vi "AB_RW_Project_Source_RESTfulVI.vi"(7 "action":T7, 8 "error in (no error)":errorcluster, 9 "index in":i32, 10 "dataSource in":T1={"RESTful VI configuration"={"Service VI Type"=enum."Web Method", "Load VI at statup"=TRUE, "Keep VI in memory"=TRUE, "Output type"=enum."Terminal", "Output format"=enum."XML", "Use headers"=TRUE, "Buffered"=TRUE, "eng_Load VI by name"=FALSE}}, 11 "buildObject":T6) -> (0 "error out":errorcluster, 1 "index out":i32, 2 "dataSource out":T1={"RESTful VI configuration"={"Service VI Type"=enum."Web Method", "Load VI at statup"=TRUE, "Keep VI in memory"=TRUE, "Output type"=enum."Terminal", "Output format"=enum."XML", "Use headers"=TRUE, "Buffered"=TRUE, "eng_Load VI by name"=FALSE}}, 3 "buildObject out":T6)   [LabVIEW 2020]
doc: "Reads and writes the data to the object property bag."
uses:
  <resource>/Framework/Providers/API/ItemRef.ctl
  <vilib>/AppBuilder/RW_Project/AB_RW_Project_PropBag_Action.ctl
  <vilib>/AppBuilder/RW_Project/AB_RW_Project_Source_RESTfulVI_Data.ctl
  <vilib>/AppBuilder/AB_Classes/Source/RESTfulVI/Configure_RESTfulVI/AB_RESTful_Configuration.ctl
  <vilib>/AppBuilder/AB_Classes/Source/RESTfulVI/Configure_RESTfulVI/AB_RESTful_VIType.ctl
  <vilib>/AppBuilder/AB_Classes/Source/RESTfulVI/Configure_RESTfulVI/AB_RESTful_OutputType.ctl
  <vilib>/AppBuilder/AB_Classes/Source/RESTfulVI/Configure_RESTfulVI/AB_RESTful_OutputFormat.ctl
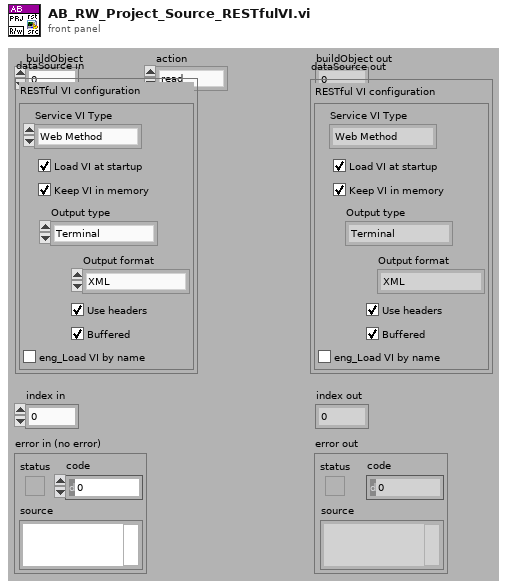
[diagram p1: front panel]
types:
  T1 = typedef "AB_RW_Project_Source_RESTfulVI_Data.ctl" = cluster{"RESTful VI configuration":T2}
  T2 = typedef "AB_RESTful_Configuration.ctl" = cluster{"Service VI Type":T3, "Load VI at statup":bool, "Keep VI in memory":bool, "Output type":T4, "Output format":T5, "Use headers":bool, "Buffered":bool, "eng_Load VI by name":bool}
  T3 = typedef "AB_RESTful_VIType.ctl" = enum32{"Web Method", "Auxiliary", "eng_Internal", "eng_Content"}
  T4 = typedef "AB_RESTful_OutputType.ctl" = enum32{"Terminal", "Stream"}
  T5 = typedef "AB_RESTful_OutputFormat.ctl" = enum32{"XML", "Text", "HTML", "JSON"}
  T6 = typedef "ItemRef.ctl" = u64
  T7 = typedef "AB_RW_Project_PropBag_Action.ctl" = enum16{"read", "write", "clear", "readPrevious", "writePrevious", "clearPrevious"}
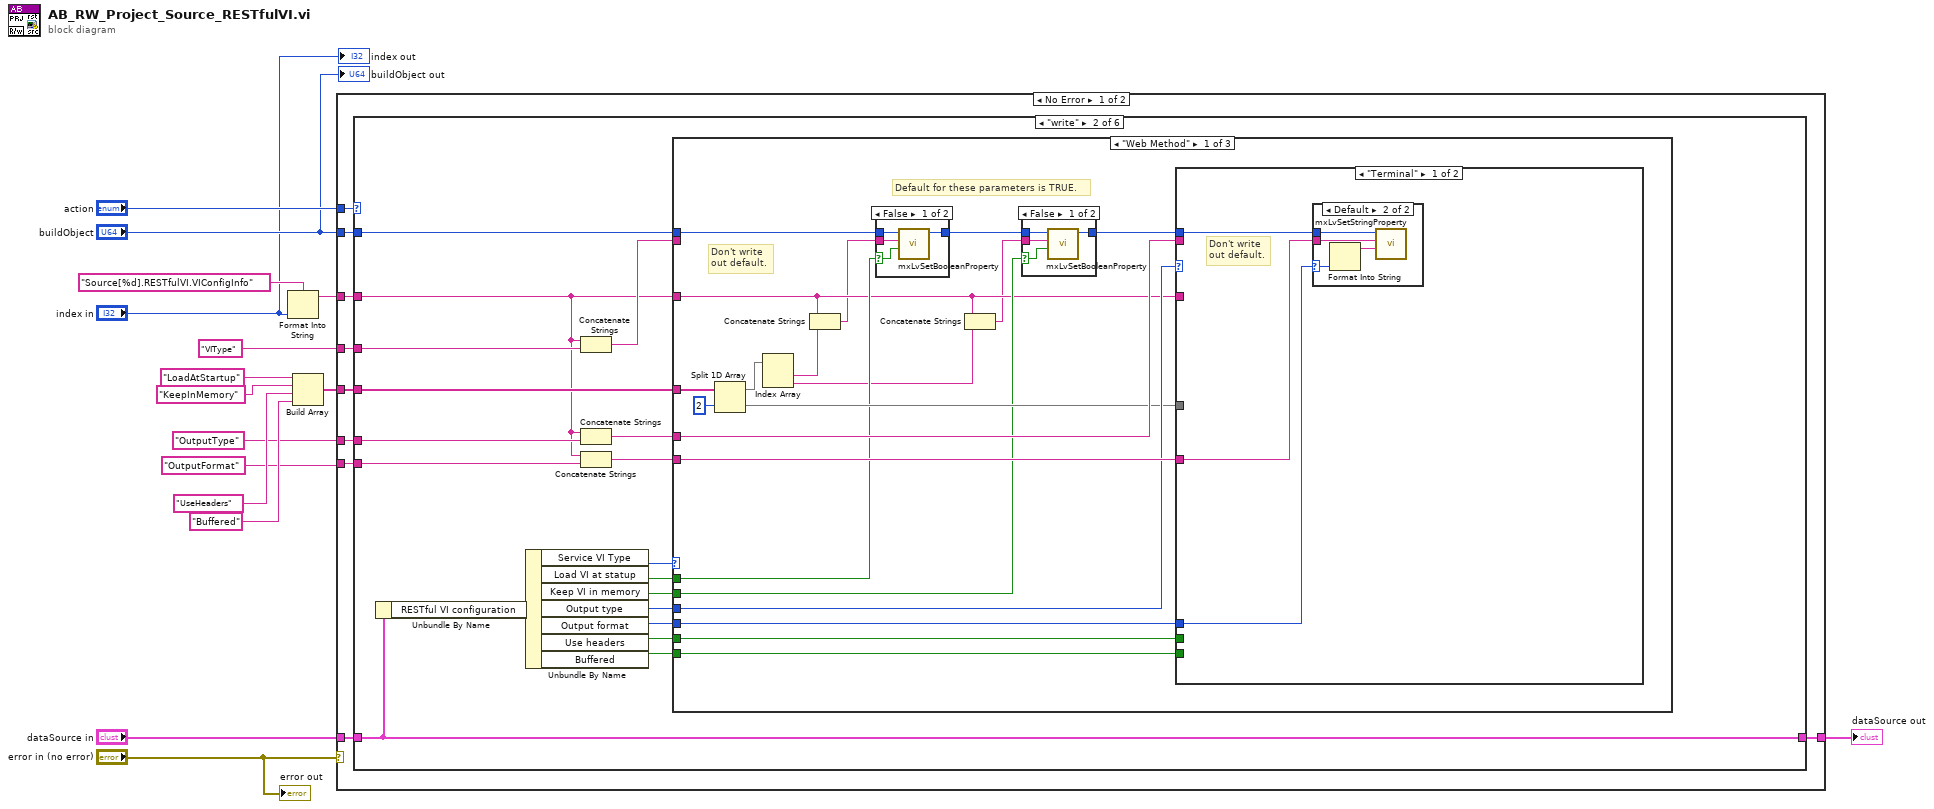
[diagram p0: block diagram]
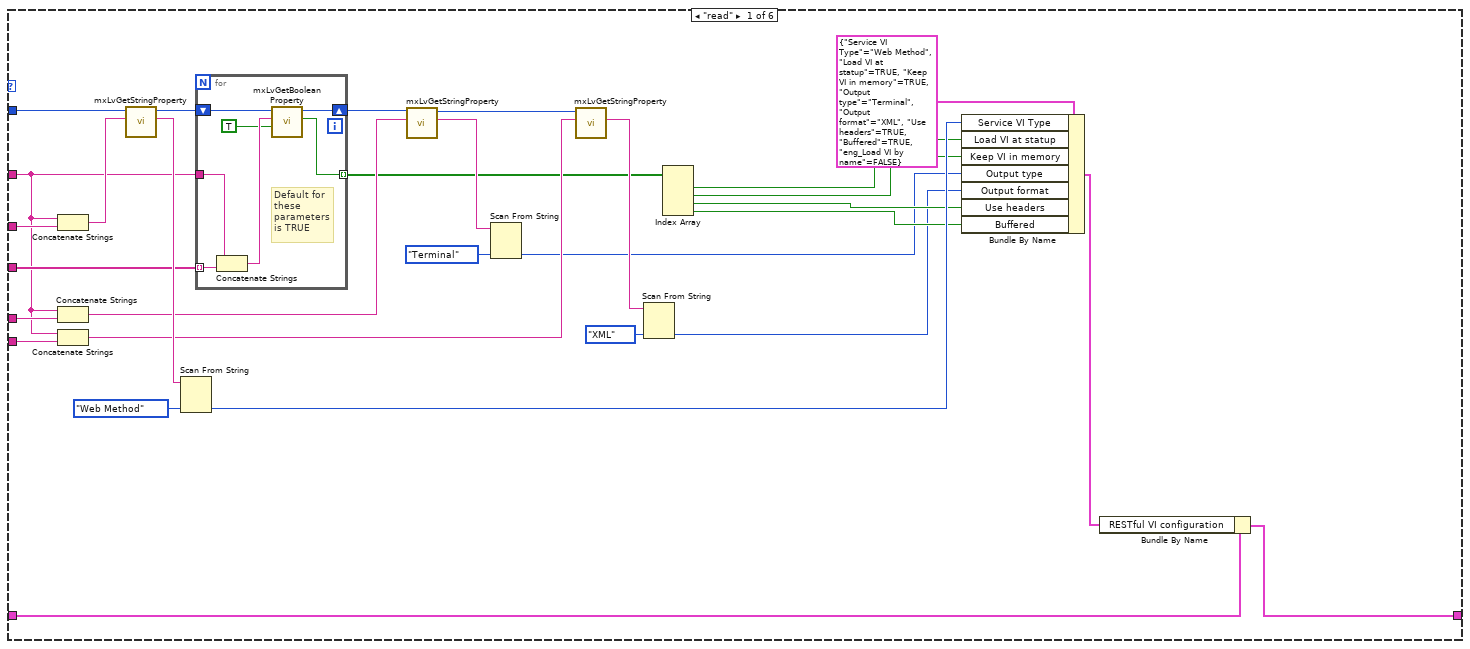
[diagram p2: hidden frame]
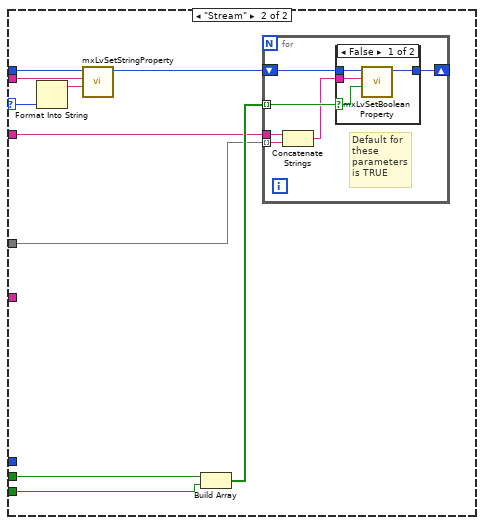
[diagram p6: hidden frame]
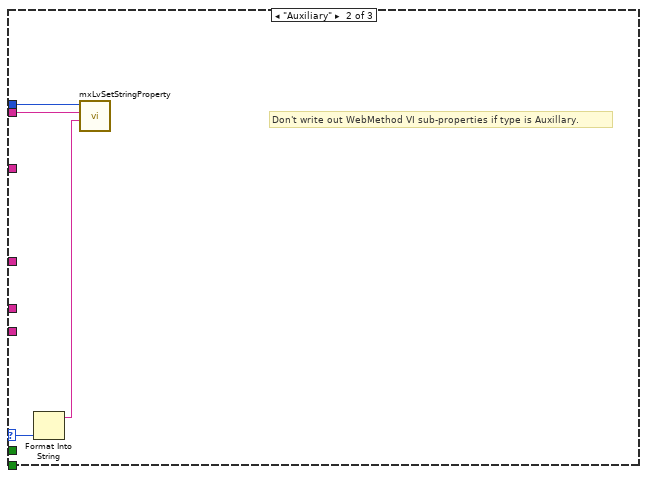
[diagram p8: hidden frame]
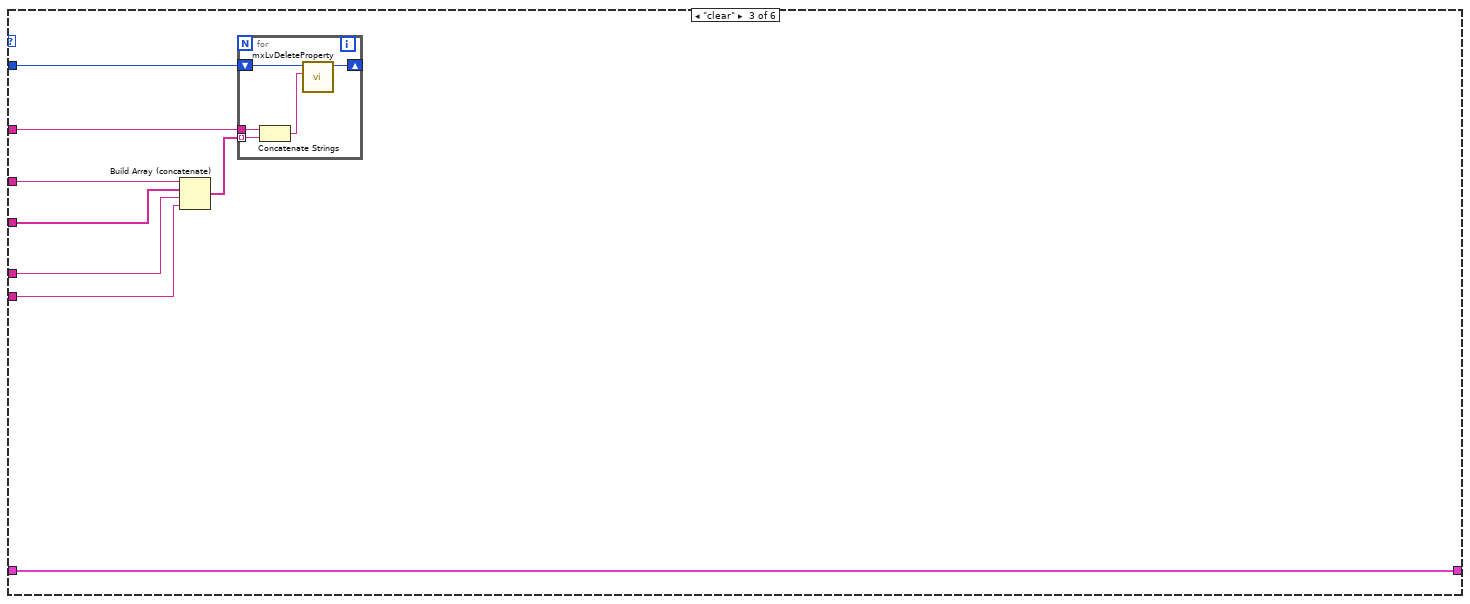
[diagram p10: hidden frame]
diagram:
  n1 = Format Into String(format string="Source[%d].RESTfulVI.VIConfigInfo", "index in") -> (resulting string=w14:string)  [unwired: 2 in, 1 out]
  n2 = Build Array("LoadAtStartup", "KeepInMemory", "UseHeaders", "Buffered") -> (w2:string[])
  n3 = case shown="No Error" "error in (no error)" {
    tunnel: "action" -> [w25 _]
    tunnel: "dataSource in" -> [w24 w159]
    tunnel: w14 -> [w23 _]
    tunnel: "buildObject" -> [w22 _]
    tunnel: [w21 w159] -> w9
    tunnel: "VIType" -> [w20 _]
    tunnel: "OutputType" -> [w19 _]
    tunnel: "OutputFormat" -> [w18 _]
    tunnel: w2 -> [w17 _]
    frame No Error {
      n4 = case shown="\"write\"" w25 {
        tunnel: w22 -> [w50 w78 w149 _ _ _]
        tunnel: w24 -> [w55 w80 w150 w156 w157 w158]
        tunnel: w23 -> [w42 w64 w144 _ _ _]
        tunnel: [w54 w80 w150 w156 w157 w158] -> w21
        tunnel: w20 -> [w51 w77 w147 _ _ _]
        tunnel: w19 -> [w43 w70 w146 _ _ _]
        tunnel: w18 -> [w41 w69 w145 _ _ _]
        tunnel: w17 -> [w45 w71 w148 _ _ _]
        frame "read" {
          n5 = Concatenate Strings(w42, w51) -> (w49:string)
          n6 = Concatenate Strings(w42, w43) -> (w39:string)
          n7 = Concatenate Strings(w42, w41) -> (w37:string)
          n8 = call <resource>:"mxLvGetStringProperty.vi"("Tag"=w49, "Item"=w50) -> ("Value"=w48:string, "Item"=w44:T6)  [unwired: 1 in, 7 out]
          n9 = Scan From String(input string=w48, default 1=AB_RESTful_VIType."Web Method" ("Service VI Type")) -> (output 1=w46:T3)  [unwired: 3 in, 3 out]
          n10 = for {
            tunnel: w45 -> [w61] mode=indexing
            tunnel: w42 -> [w62]
            shift-right: [w59] -> w40
            shift-left: w44 -> [w60]
            tunnel: [w57] -> w32 mode=indexing
            # "Default for these parameters is TRUE"
            n11 = Concatenate Strings(w62, w61) -> (w58:string)
            n12 = call <resource>:"mxLvGetBooleanProperty.vi"("Default Value (F)"=TRUE, "Tag"=w58, "Item"=w60) -> ("Value"=w57:bool, "Item"=w59:T6)  [unwired: 1 in, 6 out]
          }
          n13 = call <resource>:"mxLvGetStringProperty.vi"("Tag"=w39, "Item"=w40) -> ("Value"=w36:string, "Item"=w38:T6)  [unwired: 1 in, 7 out]
          n14 = Scan From String(input string=w36, default 1=AB_RESTful_OutputType."Terminal" ("Output type")) -> (output 1=w26:T4)  [unwired: 3 in, 3 out]
          n15 = call <resource>:"mxLvGetStringProperty.vi"("Tag"=w37, "Item"=w38) -> ("Value"=w34:string)  [unwired: 1 in, 8 out]
          n16 = Scan From String(input string=w34, default 1=AB_RESTful_OutputFormat."XML" ("Output format")) -> (output 1=w27:T5)  [unwired: 3 in, 3 out]
          n17 = Index Array(array=w32) -> (element #1=w31:bool, element #2=w30:bool, element #3=w29:bool, element #4=w28:bool)  [unwired: 4 in]
          n18 = Bundle By Name(cluster=T2 {"Service VI Type"=enum."Web Method", "Load VI at statup"=TRUE, "Keep VI in memory"=TRUE, "Output type"=enum."Terminal", "Output format"=enum."XML", "Use headers"=TRUE, "Buffered"=TRUE, "eng_Load VI by name"=FALSE} ("RESTful VI configuration"), "Service VI Type"=w46, "Load VI at statup"=w31, "Keep VI in memory"=w30, "Output type"=w26, "Output format"=w27, "Use headers"=w29, "Buffered"=w28) -> (w53:T2)
          n19 = Bundle By Name(cluster=w55, "RESTful VI configuration"=w53) -> (w54:T1)
        }
        frame "write" {
          n20 = Unbundle By Name(w80) -> ("RESTful VI configuration"=w79:T2)
          n21 = Unbundle By Name(w79) -> ("Service VI Type"=w63:T3, "Load VI at statup"=w75:bool, "Keep VI in memory"=w74:bool, "Output type"=w66:T4, "Output format"=w65:T5, "Use headers"=w73:bool, "Buffered"=w72:bool)
          n22 = Concatenate Strings(w64, w77) -> (w76:string)
          n23 = Concatenate Strings(w64, w70) -> (w68:string)
          n24 = Concatenate Strings(w64, w69) -> (w67:string)
          n25 = case shown="\"Web Method\"" w63 {
            selector: w63 -> [_ w139 _]
            tunnel: w78 -> [w91 w141 _]
            tunnel: w76 -> [_ w140 _]
            tunnel: w75 -> [w88 _ _]
            tunnel: w74 -> [w87 _ _]
            tunnel: w73 -> [w100 _ _]
            tunnel: w72 -> [w99 _ _]
            tunnel: w71 -> [w93 _ _]
            tunnel: w68 -> [w98 _ _]
            tunnel: w67 -> [w97 _ _]
            tunnel: w66 -> [w95 _ _]
            tunnel: w65 -> [w96 _ _]
            tunnel: w64 -> [w85 _ _]
            frame "Web Method" {
              # "Default for these parameters is TRUE."
              # "Don't write out default."
              n26 = Split 1D Array(array=w93, index=2) -> (first subarray=w86:string[], second subarray=w92:string[])
              n27 = Index Array(array=w86) -> (element #1=w84:string, element #2=w82:string)  [unwired: 2 in]
              n28 = Concatenate Strings(w85, w84) -> (w83:string)
              n29 = case shown="False" w88 {
                selector: w88 -> [w107 _]
                tunnel: w91 -> [w109 w110]
                tunnel: [w108 w110] -> w90
                tunnel: w83 -> [w106 _]
                frame False {
                  n30 = call <resource>:"mxLvSetBooleanProperty.vi"("Value (F)"=w107, "Tag"=w106, "Item"=w109) -> ("Item"=w108:T6)  [unwired: 2 in, 6 out]
                }
                frame True {
                }
              }
              n31 = Concatenate Strings(w85, w82) -> (w81:string)
              n32 = case shown="False" w87 {
                selector: w87 -> [w102 _]
                tunnel: w90 -> [w104 w105]
                tunnel: [w103 w105] -> w89
                tunnel: w81 -> [w101 _]
                frame False {
                  n33 = call <resource>:"mxLvSetBooleanProperty.vi"("Value (F)"=w102, "Tag"=w101, "Item"=w104) -> ("Item"=w103:T6)  [unwired: 2 in, 6 out]
                }
                frame True {
                }
              }
              n34 = case shown="\"Terminal\"" w95 {
                selector: w95 -> [_ w118]
                tunnel: w100 -> [_ w127]
                tunnel: w99 -> [_ w126]
                tunnel: w92 -> [_ w124]
                tunnel: w98 -> [_ w122]
                tunnel: w97 -> [w113 _]
                tunnel: w96 -> [w112 _]
                tunnel: w85 -> [_ w121]
                tunnel: w89 -> [w111 w120]
                frame "Terminal" {
                  # "Don't write out default."
                  n35 = case shown="Default" w112 {
                    selector: w112 -> [_ w114]
                    tunnel: w111 -> [_ w117]
                    tunnel: w113 -> [_ w115]
                    frame "XML" {
                    }
                    frame Default {
                      n36 = Format Into String(w114) -> (resulting string=w116:string)  [unwired: 3 in, 1 out]
                      n37 = call <resource>:"mxLvSetStringProperty.vi"("Value (\"\")"=w116, "Tag"=w115, "Item"=w117) -> ()  [unwired: 2 in, 7 out]
                    }
                  }
                }
                frame "Stream" {
                  n38 = Format Into String(w118) -> (resulting string=w119:string)  [unwired: 3 in, 1 out]
                  n39 = call <resource>:"mxLvSetStringProperty.vi"("Value (\"\")"=w119, "Tag"=w122, "Item"=w120) -> ("Item"=w123:T6)  [unwired: 2 in, 6 out]
                  n40 = Build Array(w127, w126) -> (w125:bool[])
                  n41 = for {
                    shift-right: [w132] -> _
                    shift-left: w123 -> [w133]
                    tunnel: w125 -> [w131] mode=indexing
                    tunnel: w124 -> [w129] mode=indexing
                    tunnel: w121 -> [w130]
                    # "Default for these parameters is TRUE"
                    n42 = Concatenate Strings(w130, w129) -> (w128:string)
                    n43 = case shown="False" w131 {
                      selector: w131 -> [w134 _]
                      tunnel: w133 -> [w137 w138]
                      tunnel: w128 -> [w136 _]
                      tunnel: [w135 w138] -> w132
                      frame False {
                        n44 = call <resource>:"mxLvSetBooleanProperty.vi"("Value (F)"=w134, "Tag"=w136, "Item"=w137) -> ("Item"=w135:T6)  [unwired: 2 in, 6 out]
                      }
                      frame True {
                      }
                    }
                  }
                }
              }
            }
            frame "Auxiliary" {
              # "Don't write out WebMethod VI sub-properties if type is Auxillary."
              n45 = Format Into String(w139) -> (resulting string=w142:string)  [unwired: 3 in, 1 out]
              n46 = call <resource>:"mxLvSetStringProperty.vi"("Value (\"\")"=w142, "Tag"=w140, "Item"=w141) -> ()  [unwired: 2 in, 7 out]
            }
            frame "eng_Internal", "eng_Content" {
              # "Internal and Content VIs are only added during build and should not be saved."
            }
          }
        }
        frame "clear" {
          n47 = Build Array (concatenate)(w147, w148, w146, w145) -> (w143:string[])
          n48 = for {
            shift-right: [w154] -> _
            shift-left: w149 -> [w155]
            tunnel: w144 -> [w153]
            tunnel: w143 -> [w152] mode=indexing
            n49 = Concatenate Strings(w153, w152) -> (w151:string)
            n50 = call <resource>:"mxLvDeleteProperty.vi"("Tag"=w151, "Item"=w155) -> ("Item"=w154:T6)  [unwired: 2 in, 7 out]
          }
        }
        frame "readPrevious" {
        }
        frame "writePrevious" {
        }
        frame "clearPrevious" {
        }
      }
    }
    frame Error {
    }
  }
  "dataSource out" <- w9
  "error out" <- "error in (no error)"
  "buildObject out" <- "buildObject"
  "index out" <- "index in"
